vi "upper.vi"() -> ()   [LabVIEW 2022 SP3]
panel:
  out "Output":string
  in  "Input":string
  # "What do you think about ECE 144?"
  # "(UPPERCASE output)"
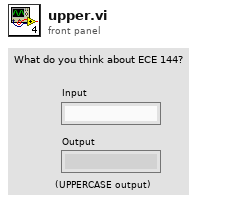
[diagram p1: front panel]
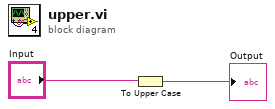
[diagram p0: block diagram]
diagram:
  n1 = To Upper Case(1:"Input") -> (0:→"Output":string)
